vi "Close FIFOs.vi"(8 "error in (no error)":errorcluster, 11 "RT Data in":T1 {"Channels"."Voltage"."Ref"."Data Reference" format="%.0x"; "Channels"."Current"."Ref"."Data Reference" format="%.0x"; "Channels"."Read Volt"."Ref" format="%.0x"; "Channels"."Mode"."Ref" format="%.0x"}) -> (0 "error out":errorcluster, 3 "RT Data out":T1 {"Channels"."Voltage"."Ref"."Data Reference" format="%.0x"; "Channels"."Current"."Ref"."Data Reference" format="%.0x"; "Channels"."Read Volt"."Ref" format="%.0x"; "Channels"."Mode"."Ref" format="%.0x"})   [LabVIEW 2011, in "Switch-DMM Custom Device.lvlib"]
uses:
  Switch-DMM Custom Device.lvlib
  Controls/RT Data.ctl
  Controls/Channels.ctl
  Controls/Single Channel.ctl
  <vilib>/NI Veristand/Custom Device API/Data Reference.ctl
  Controls/Block Channels.ctl
  <vilib>/NI Veristand/Custom Device API/Block Data Reference.ctl
  Controls/Communication.ctl
  Controls/Async Status.ctl
  Controls/Async State.ctl
  Controls/Async Command.ctl
  Controls/Async Events.ctl
  <vilib>/NI Veristand/Custom Device API/Custom Device API.lvlib
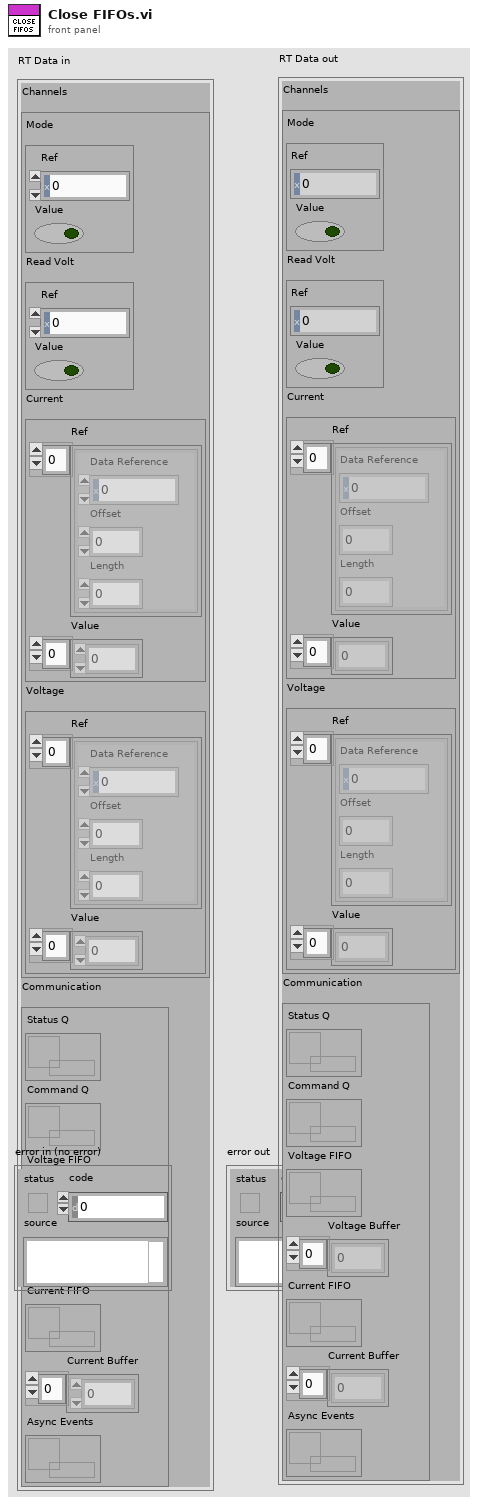
[diagram p1: front panel]
types:
  T1 = typedef "Switch-DMM Custom Device.lvlib/RT Data.ctl" = cluster{"Channels":T2, "Communication":T7}
  T2 = typedef "Switch-DMM Custom Device.lvlib/Channels.ctl" = cluster{"Mode":T3, "Read Volt":T3, "Current":T5, "Voltage":T5}
  T3 = typedef "Switch-DMM Custom Device.lvlib/Single Channel.ctl" = cluster{"Ref":T4, "Value":bool}
  T4 = typedef "Custom Device API.lvlib/Data Reference.ctl" = i32
  T5 = typedef "Switch-DMM Custom Device.lvlib/Block Channels.ctl" = cluster{"Ref":T6[], "Value":dbl[]}
  T6 = typedef "Custom Device API.lvlib/Block Data Reference.ctl" = cluster{"Data Reference":T4, "Offset":i32, "Length":i32}
  T7 = typedef "Switch-DMM Custom Device.lvlib/Communication.ctl" = cluster{"Status Q":refnum<queue>, "Command Q":refnum<queue>, "Voltage FIFO":refnum<k33>, "Voltage Buffer":dbl[], "Current FIFO":refnum<k33>, "Current Buffer":dbl[], "Async Events":refnum<queue>}
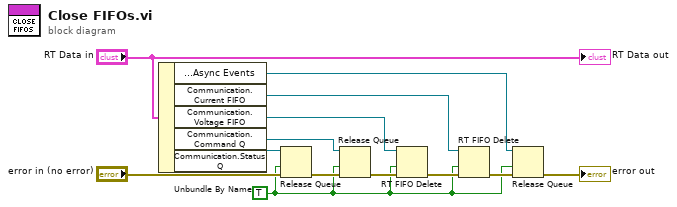
[diagram p0: block diagram]
diagram:
  w1 = TRUE ("force destroy? (F)")
  n1 = Unbundle By Name("RT Data in") -> ("Communication.Async Events"=w5:refnum<queue>, "Communication.Current FIFO"=w3:refnum<k33>, "Communication.Voltage FIFO"=w4:refnum<k33>, "Communication.Command Q"=w9:refnum<queue>, "Communication.Status Q"=w13:refnum<queue>)
  n2 = Release Queue(queue=w13, force destroy? (F)=w1, error in (no error)="error in (no error)") -> (error out=w12:errorcluster)  [unwired: 2 out]
  n3 = Release Queue(queue=w9, force destroy? (F)=w1, error in (no error)=w12) -> (error out=w8:errorcluster)  [unwired: 2 out]
  n4 = RT FIFO Delete(0:w4, 2:w1, 3:w8) -> (11:w7:errorcluster)
  n5 = RT FIFO Delete(0:w3, 2:w1, 3:w7) -> (11:w6:errorcluster)
  n6 = Release Queue(queue=w5, force destroy? (F)=w1, error in (no error)=w6) -> (error out=→"error out":errorcluster)  [unwired: 2 out]
  "RT Data out" <- "RT Data in"
